vi "Update Connection Configuration.vi"(0 "Data Value Reference in":refnum<data-value>, 5 "Connection Type":T2, 7 "Configuration":T1={"Configuration ID"="", "HTTP"={"Verify Server?"=TRUE, "Server URL"="", "CA Certificate File"="", "User Info"={"Username"="", "Password"=""}, "API Key"=""}}, 11 "error in":errorcluster) -> (15 "error out":errorcluster)   [LabVIEW 2015, in "SystemLink File editor node.lvclass"]
doc: "Update the \"Connection Configuration\" cluster of the corresponding \"SystemLink Tag Module Configuration.lvclass\""
uses:
  SystemLink File editor node.lvclass
  module/configuration/Connection Type.ctl
  <vilib>/NI/DCAF/Tag Editor Core/Configuration Editor/Classes/Module editor node/module editor node.lvclass
  SystemLink File editor node.lvclass/SystemLink File editor node.ctl
  module/configuration/Connection Configuration.ctl
  module/configuration/SystemLink File configuration.lvclass/SystemLink File configuration.ctl
  module/configuration/Write Connection Configuration.vi
  module/configuration/SystemLink File configuration.lvclass
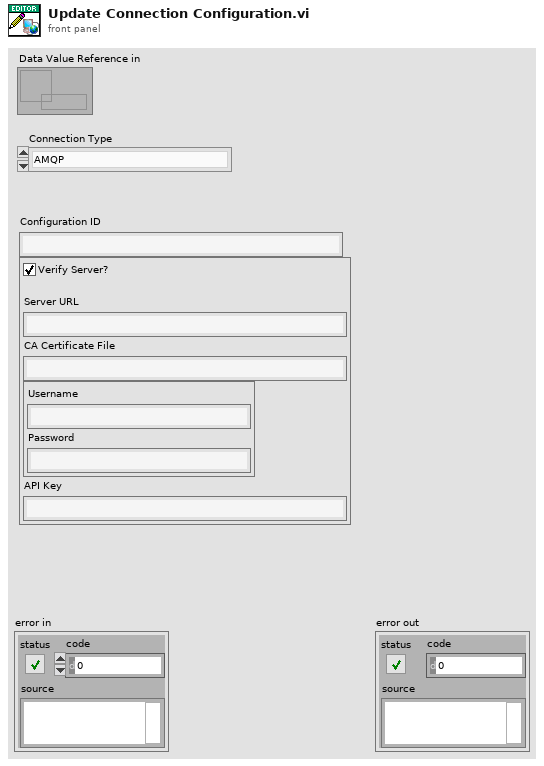
[diagram p1: front panel]
types:
  T1 = cluster{"Configuration ID":string, "HTTP":cluster{"Verify Server?":bool, "Server URL":string, "CA Certificate File":string, "User Info":cluster{"Username":string, "Password":string}, "API Key":string}}
  T2 = typedef "SystemLink File configuration.lvclass/Connection Type.ctl" = enum16{"AMQP", "HTTP", "API Key (SystemLink Cloud)"}
  T3 = cluster{"Verify Server?":bool, "Server URL":string, "CA Certificate File":string, "User Info":cluster{"Username":string, "Password":string}, "API Key":string}
  T4 = typedef "SystemLink File configuration.lvclass/Connection Configuration.ctl" = cluster{"Connection Type":T2, "AMQP":cluster{"Configuration ID":string}, "HTTP":cluster{"Verify Server?":bool, "Server URL":string, "CA Certificate File":string, "User Info":cluster{"Username":string, "Password":string}, "API Key":string}}
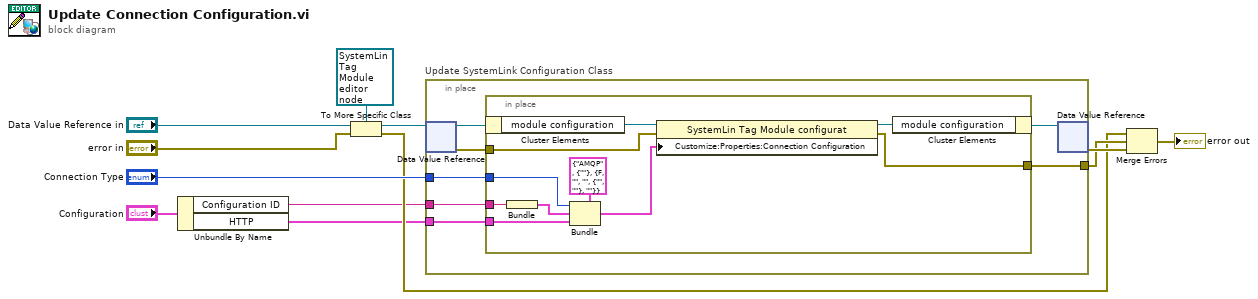
[diagram p0: block diagram]
diagram:
  n1 = Unbundle By Name("Configuration") -> ("Configuration ID"=w1:string, "HTTP"=w2:T3)
  n2 = To More Specific Class(target class=refnum<data-value> refnum ("Data Value Reference in"), reference="Data Value Reference in", error in="error in") -> (specific class reference=w11:refnum<data-value>, error out=w4:errorcluster)
  n3 = in-place "Update SystemLink Configuration Class" {
    in-place-border: "Connection Type" -> [w15]
    in-place-border: w1 -> [w16]
    in-place-border: w2 -> [w17]
    in-place-border: [w13] -> w5
    n4 = in-place-dvr #1(w11) -> (w19:refnum<class "SystemLink File editor node.lvclass">, w14:errorcluster)
    n5 = in-place {
      in-place-border: w17 -> [w23]
      in-place-border: w16 -> [w27]
      in-place-border: w15 -> [w25]
      in-place-border: w14 -> [w21]
      in-place-border: [w20] -> w13
      n6 = in-place-cluster #2(w19) -> ("module configuration"=w29:refnum<class "SystemLink File configuration.lvclass">)
      n7 = Bundle("Configuration ID"=w27) -> (w24:cluster{"Configuration ID":string})  [unwired: 1 in]
      n8 = Bundle(cluster=T4 {"Connection Type"=enum."AMQP", "AMQP"={"Configuration ID"=""}, "HTTP"={"Verify Server?"=FALSE, "Server URL"="", "CA Certificate File"="", "User Info"={"Username"="", "Password"=""}, "API Key"=""}} ("Connection Configuration"), "Connection Type"=w25, "AMQP"=w24, "HTTP"=w23) -> (w22:T4)
      n9 = property class="SystemLin Tag Module configurat"(reference=w29, error in=w21, "Customize:Properties:Connection Configuration"=w22) -> (reference out=w28:refnum<class "SystemLink File configuration.lvclass">, error out=w20:errorcluster)
      n10 = in-place-cluster #2("module configuration"=w28) -> (w18:refnum<class "SystemLink File editor node.lvclass">)
    }
    n11 = in-place-dvr #1(w18) -> (w6:errorcluster)  [unwired: 1 out]
  }
  n12 = Merge Errors(w4, w5, w6) -> (→"error out":errorcluster)
